vi "ATS_SetRecord.vi"(10 "RecordIn":T1={"Count"=1, "Presize"=1, "Length"=0}, 11 "DeviceIn":i32) -> (0 "Return Code":u32, 2 "RecordOut":T1={"Count"=1, "Presize"=1, "Length"=0}, 3 "DeviceOut":i32)   [LabVIEW 2014]
doc: "_____AlazarTech, Scope_____\n\nConfigure the number of records for the device to capture."
uses:
  ATS_ctl/Record.ctl
  ATS_ctl/ATS_Global_Ctrl.ctl
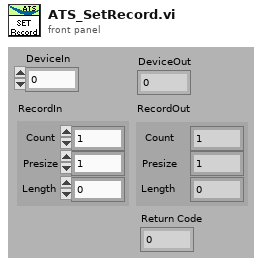
[diagram p1: front panel]
types:
  T1 = typedef "Record.ctl" = cluster{"Count":u32, "Presize":u32, "Length":u32}
  T2 = typedef "ATS_Global_Ctrl.ctl" = enum16{"Init_Device", "Clear_ALL", "Set", "Get"}
  T3 = typedef "ATS_Global_Specs_Ctrl.ctl" = cluster{"ClckSource":cluster{"Internal":bool, "External":bool, "Medium Ext.":bool, "Slow Ext.":bool, "Ext. AC":bool, "Ext. DC":bool, "Ext. (PLL)":bool}, "ClckRate":cluster{"1 kS/s":bool, "2 kS/s":bool, "5 kS/s":bool, "10 kS/s":bool, "20 kS/s":bool, "50 kS/s":bool, "100 kS/s":bool, "200 kS/s":bool, "500 kS/s":bool, "1 MS/s":bool, "2 MS/s":bool, "5 MS/s":bool, "10 MS/s":bool, "20 MS/s":bool, "25 MS/s":bool, "50 MS/s":bool, "100 MS/s":bool, "125 MS/s":bool, "160 MS/s":bool, "180 MS/s":bool, "200 MS/s":bool, "250 MS/s":bool, "500 MS/s":bool, "1 GS/s":bool}, "ClckEdge":cluster{"Rising":bool, "Falling":bool}, "InputCoupling":cluster{"AC":bool, "DC":bool}, "InputRange":cluster{"20mV":bool, "40mV":bool, "50mV":bool, "80mV":bool, "100mV":bool, "200mV":bool, "400mV":bool, "500mV":bool, "800mV":bool, "1 V":bool, "2 V":bool, "4 V":bool, "5 V":bool, "8 V":bool, "10 V":bool, "16 V":bool, "20 V":bool, "40 V":bool, "HiFi":bool, "1.25 V":bool}, "Impedance":cluster{"1M ohms":bool, "50 ohms":bool, "300 ohms":bool}, "Bandwidth":cluster{"Full":bool, "Reduce":bool}, "RangeLim(50)":string, "AsyncDMA":cluster{"OnBoard":bool, "FPGA":bool}, "Memory":cluster{"VerifMem":bool, "HighMem":bool, "Combine":bool, "HighRecord":bool}, "ExtTrigCoupling":cluster{"AC":bool, "DC":bool}, "ExtTrigRange":cluster{"1 V":bool, "5 V":bool, "\nTTL":bool}, "AUX_IO_Trig":cluster{"Trig_Out":bool, "Trig_In":bool}, "AUX_IO_Slope":cluster{"Rising":bool, "Falling":bool}, "MaxPretrig":cluster{"MEM":u32, "FIFO":u32}, "AUX_I/O_Trig":cluster{"OUT_Trigger":bool, "OUT_PACER":bool, "OUT_BUSY":bool, "OUT_CLOCK":bool, "OUT_RESERVED":bool, "OUT_CAPTURE_ALMOST_DONE":bool, "OUT_AUXILIARY":bool, "OUT_SERIAL_DATA":bool, "IN_TRIGGER_ENABLE":bool, "IN_DIGITAL_TRIGGER":bool, "IN_GATE":bool, "IN_CAPTURE_ON_DEMAND":bool, "IN_RESET_TIMESTAMP":bool, "IN_SLOW_EXTERNAL_CLOCK":bool, "INPUT_AUXILIARY":bool, "INPUT_SERIAL_DATA":bool}, "ChannelsPerBoard":u8}
  T4 = typedef "ATS_Set_Value.ctl" = cluster{"Clock (s)":dbl, "RangeA (v)":dbl, "RangeB (v)":dbl, "Ranges (v)":dbl[]}
  T5 = typedef "ATS_Global_4Ch.ctl" = cluster{"Record":T1, "Clock":T6, "Inputs":T10, "Trigger":T16}
  T6 = typedef "Clock.ctl" = cluster{"ClckSource":T7, "ClckRate":T8, "ClckEdge":T9, "Decimation":u32}
  T7 = typedef "ClockSource.ctl" = enum16{"Internal", "External", "Medium Ext.", "Slow Ext.", "Ext. AC", "Ext. DC", "Ext. (PLL)"}
  T8 = typedef "ClockRate.ctl" = u32
  T9 = typedef "ClockEdge.ctl" = u16
  T10 = typedef "ATS_InputArray.ctl" = T11[]
  T11 = typedef "InputCtrl.ctl" = cluster{"Coupling":T12, "Range":T13, "Impedance":T14, "Bandwidth":T15}
  T12 = typedef "Coupling.ctl" = enum16{"AC", "DC"}
  T13 = typedef "Range.ctl" = u32
  T14 = typedef "Impedance.ctl" = enum16{"1M ohms", "50 ohms"}
  T15 = typedef "Bandwidth.ctl" = enum16{"Full Bandwidth", "Reduce Bandwidth"}
  T16 = typedef "ATS_Trigger_4Ch.ctl" = cluster{"TrigOperation":T17, "Timeout (s)":dbl, "Trig. Delay":u32, "Engine X":T18, "Engine Y":T18, "ExtTrigControl":T20}
  T17 = typedef "TriggerOperation.ctl" = enum16{"Only X", "Only Y", "X or Y", "X and Y", "X xor Y", "X and not Y", "not X and Y"}
  T18 = typedef "ATS_TriggerEngine_4Ch.ctl" = cluster{"Source":T19, "Slope":enum32{"Positive", "Negative"}, "Level":u32}
  T19 = typedef "ATS_TriggerSource_4Ch.ctl" = enum32{"Chan_A", "Chan_B", "External", "Disable", "Chan_C", "Chan_D"}
  T20 = typedef "ExtTrigger.ctl" = cluster{"Coupling":T12, "Range":T21}
  T21 = typedef "ExtTrigRange.ctl" = enum16{"1 V", "5 V", "TTL"}
  T22 = typedef "Device_Info.ctl" = cluster{"Handle":u32, "Board":string, "CPLD":string, "MemorySize":u32, "SampleSize":u8, "ID":i32, "High_Memory":bool, "Chan/Board":u8}
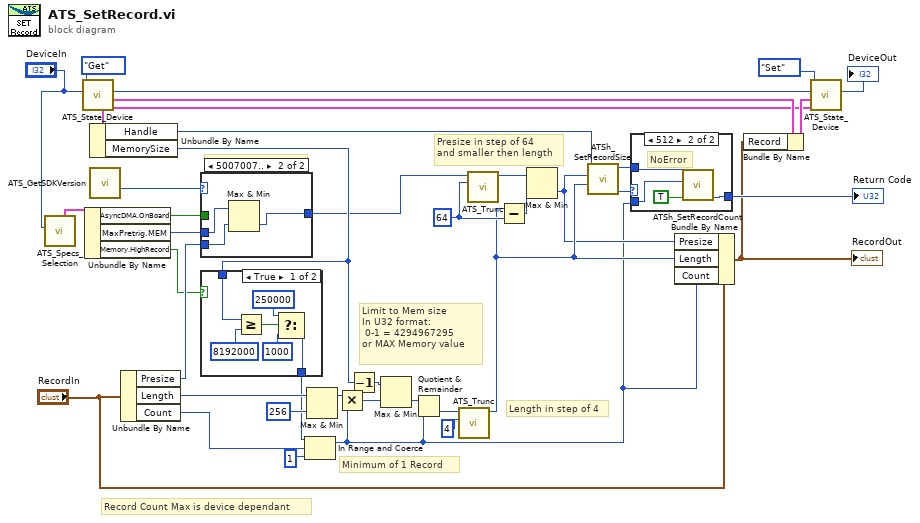
[diagram p0: block diagram]
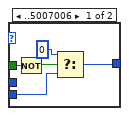
[diagram p2: hidden frame]
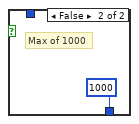
[diagram p3: hidden frame]
diagram:
  w30 = u32 64 ("TruncValue")
  # "ATSApi dependant"
  # "Record Count Max is device dependant"
  # "Minimum of 1 Record"
  # "Limit to Mem size\nIn U32 format:  \n 0-1 = 4294967295 \nor MAX Memory value"
  # "Presize in step of 64\nand smaller then length"
  # "Length in step of 4"
  n1 = call "ATS_Specs_Selection.vi"("Device"="DeviceIn") -> ("Specifications"=w3:T3)  [unwired: 4 in, 6 out]
  n2 = call "ATS_State_Device.vi"("DeviceIn"="DeviceIn", "ATS_GBL_Ctrl"=ATS_Global_Ctrl."Get") -> ("Ref_Out"=w15:T4, "SetupOut"=w17:T5, "DeviceOut"=w26:i32, "DevInfo_Out"=w16:T22)  [unwired: 4 in, 2 out]
  n3 = Unbundle By Name(w3) -> ("AsyncDMA.OnBoard"=w7:bool, "MaxPretrig.MEM"=w6:u32, "Memory.HighRecord"=w2:bool)
  n4 = Unbundle By Name(w16) -> ("Handle"=w36:u32, "MemorySize"=w10:u32)
  n5 = call "ATS_GetSDKVersion.vi"() -> ("SDK_#"=w1:u32)  [unwired: 9 in, 2 out]
  n6 = Unbundle By Name("RecordIn") -> ("Presize"=w4:u32, "Length"=w14:u32, "Count"=w19:u32)
  n7 = case shown="5007007.." w1 {
    tunnel: w7 -> [w43 _]
    tunnel: w4 -> [w42 w47]
    tunnel: [w41 w46] -> w5
    tunnel: w6 -> [_ w48]
    frame ..5007006 {
      n8 = Not(x=w43) -> (.not. x?=w44:bool)
      n9 = Select(t=u32 0 ("Presize"), s=w44, f=w42) -> (s? t:f=w41:u32)
    }
    frame 5007007.. {
      n10 = Max & Min(x=w48, y=w47) -> (min(x,y)=w46:u32)  [unwired: 1 out]
    }
  }
  n11 = case shown="True" w2 {
    tunnel: [w50 u32 1000 ("upper limit")] -> w9
    tunnel: w10 -> [w54 _]
    frame True {
      n12 = Greater Or Equal?(x=w54, y=u32 8192000) -> (x >= y?=w49:bool)
      n13 = Select(t=u32 250000 ("upper limit"), s=w49, f=u32 1000 ("upper limit")) -> (s? t:f=w50:u32)
    }
    frame False {
      # "Max of 1000"
    }
  }
  n14 = In Range and Coerce(upper limit=w9, x=w19, lower limit=u32 1 ("y")) -> (coerced(x)=w21:u32)  [unwired: 1 out]
  n15 = Max & Min(x=w14, y=u32 256) -> (max(x,y)=w13:u32)  [unwired: 1 out]
  n16 = Multiply(x=w13, y=w21) -> (x*y=w35:u32)
  n17 = Decrement(x=w10) -> (x-1=w11:u32)
  n18 = Max & Min(x=w11, y=w35) -> (min(x,y)=w34:u32)  [unwired: 1 out]
  n19 = Quotient & Remainder(x=w34, y=w21) -> (floor(x/y)=w32:u32)  [unwired: 1 out]
  n20 = call "ATS_Trunc.vi"("TruncValue"=u32 4, "Value"=w32) -> ("NewValue"=w23:u32)  [unwired: 5 in]
  n21 = call "ATS_Trunc.vi"("TruncValue"=w30, "Value"=w5) -> ("NewValue"=w31:u32)  [unwired: 5 in]
  n22 = Subtract(x=w23, y=w30) -> (x-y=w29:u32)
  n23 = Max & Min(x=w31, y=w29) -> (min(x,y)=w22:u32)  [unwired: 1 out]
  n24 = call "ATSh_SetRecordSize.vi"("Length"=w23, "Presize"=w22, "HandleIn"=w36) -> ("Return Code"=w39:u32, "HandleOut"=w40:u32)  [unwired: 7 in]
  n25 = case shown="512" w39 {
    selector: w39 -> [w56 _]
    tunnel: w21 -> [_ w60]
    tunnel: w40 -> [_ w59]
    tunnel: [w56 w58] -> w38
    frame 0, Default {
      # "Error"
    }
    frame 512 {
      # "NoError"
      n26 = call "ATSh_SetRecordCount.vi"("NoLimit (T)"=TRUE ("DMA (F)"), "#Record"=w60, "HandleIn"=w59) -> ("Return Code"=w58:u32)  [unwired: 7 in, 1 out]
    }
  }
  "Return Code" <- w38
  n27 = Bundle By Name(cluster="RecordIn", "Presize"=w22, "Length"=w23, "Count"=w21) -> (w25:T1)
  "RecordOut" <- w25
  n28 = Bundle By Name(cluster=w17, "Record"=w25) -> (w18:T5)
  n29 = call "ATS_State_Device.vi"("Ref_In"=w15, "SetupIn"=w18, "DeviceIn"=w26, "ATS_GBL_Ctrl"=ATS_Global_Ctrl."Set") -> ("DeviceOut"=→"DeviceOut":i32)  [unwired: 2 in, 5 out]
